vi "Disabled Property(Main Controls)_Abort.vi"(8 "error in (no error)":errorcluster, 11 "MWWL Verification in":refnum<class "MWWL Verification.lvclass">) -> (0 "error out":errorcluster, 3 "MWWL Verification out":refnum<class "MWWL Verification.lvclass">)   [LabVIEW 2018, in "MWWL Verification.lvlib" / "MWWL Verification.lvclass"]
uses:
  MWWL Verification.lvclass
  MWWL Verification.lvclass/MWWL Verification.ctl
types:
  T1 = enum8{"Enabled", "Disabled", "Disabled and Grayed Out"}
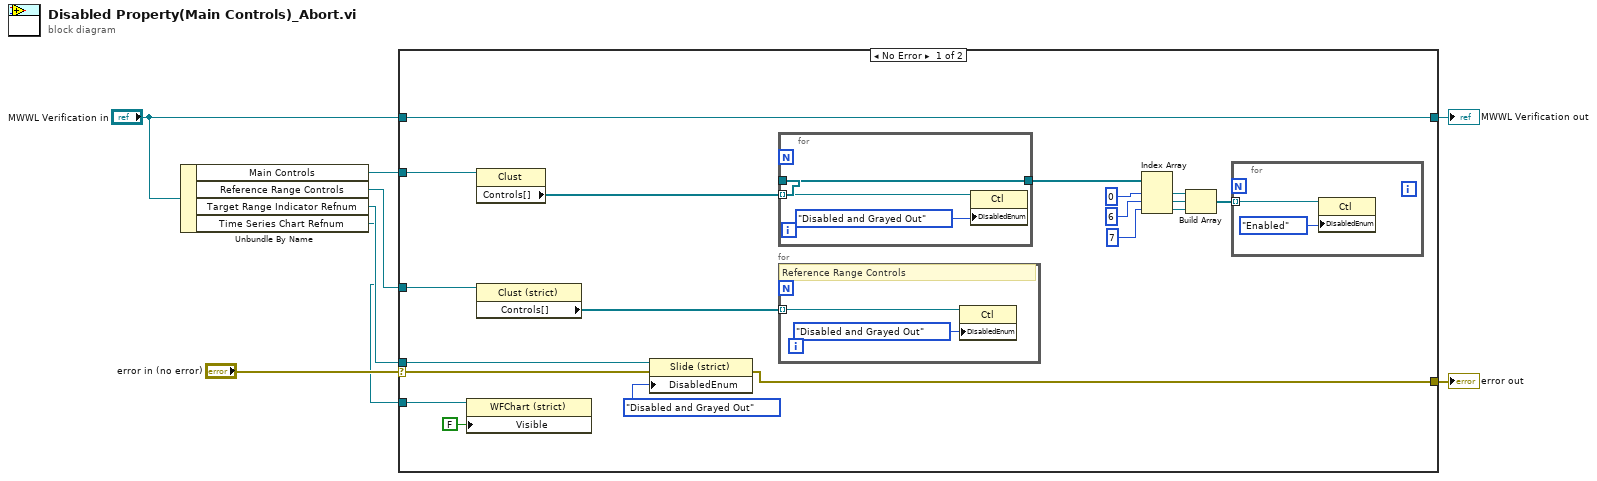
[diagram p0: block diagram]
diagram:
  n1 = Unbundle By Name("MWWL Verification in") -> ("Main Controls"=w4:refnum<vi>, "Reference Range Controls"=w3:refnum<vi>, "Target Range Indicator Refnum"=w2:refnum<vi>, "Time Series Chart Refnum"=w1:refnum<vi>)
  n2 = case shown="No Error" "error in (no error)" {
    selector: "error in (no error)" -> [w11 w36]
    tunnel: [w15 w36] -> w7
    tunnel: [w27 w35] -> w6
    tunnel: "MWWL Verification in" -> [w27 w35]
    tunnel: w4 -> [w26 _]
    tunnel: w3 -> [w25 _]
    tunnel: w2 -> [w12 _]
    tunnel: w1 -> [w10 _]
    frame No Error {
      n3 = property class="WFChart (strict)"(reference=w10, "Visible"=FALSE) -> ()  [unwired: 1 in, 2 out]
      n4 = property class="Clust"(reference=w26) -> ("Controls[]"=w21:refnum<vi>[])  [unwired: 1 in, 2 out]
      n5 = property class="Clust (strict)"(reference=w25) -> ("Controls[]"=w24:refnum<vi>[])  [unwired: 1 in, 2 out]
      n6 = property class="Slide (strict)"(reference=w12, error in=w11, "DisabledEnum"=T1."Disabled and Grayed Out" ("Disabled")) -> (error out=w15:errorcluster)  [unwired: 1 out]
      n7 = for {
        tunnel: w21 -> [w31] mode=indexing
        tunnel: [w30] -> w20
        tunnel: w21 -> [w30]
        n8 = property class="Ctl"(reference=w31, "DisabledEnum"=T1."Disabled and Grayed Out" ("Disabled")) -> ()  [unwired: 1 in, 2 out]
      }
      n9 = for {
        tunnel: w24 -> [w33] mode=indexing
        # "Reference Range Controls"
        n10 = property class="Ctl"(reference=w33, "DisabledEnum"=T1."Disabled and Grayed Out" ("Disabled")) -> ()  [unwired: 1 in, 2 out]
      }
      n11 = Index Array(array=w20, index #1=0 ("index"), index #2=6 ("index"), index #3=7 ("index")) -> (element #1=w19:refnum<vi>, element #2=w18:refnum<vi>, element #3=w17:refnum<vi>)
      n12 = Build Array(w19, w18, w17) -> (w16:refnum<vi>[])
      n13 = for {
        tunnel: w16 -> [w28] mode=indexing
        n14 = property class="Ctl"(reference=w28, "DisabledEnum"=T1."Enabled" ("Disabled")) -> ()  [unwired: 1 in, 2 out]
      }
    }
    frame Error {
    }
  }
  "error out" <- w7
  "MWWL Verification out" <- w6
